vi "BRig_RT__Case_Exp__State_start__sendExpData_saveData.vi"(10 "input_dataLC":u16[](array[numeric]), 11 "input_dataExp":u16[](array[numeric])) -> ()   [LabVIEW 2014]
uses:
  <vilib>/Utility/file.llb/Write To Spreadsheet File (DBL).vi
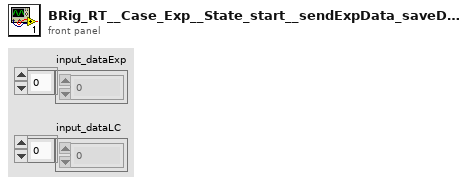
[diagram p1: front panel]
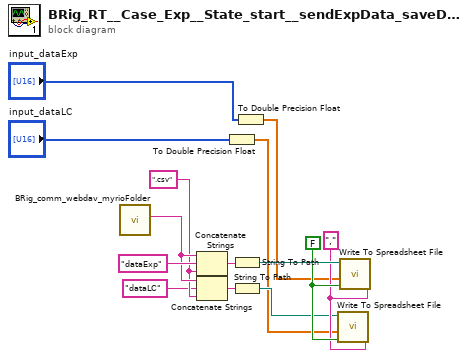
[diagram p0: block diagram]
diagram:
  w6 = "," ("delimiter (\\t)")
  w7 = FALSE ("append to file? (new file:F)")
  w10 = ".csv" ("string")
  n1 = call "BRig_comm_webdav_myrioFolder.vi"() -> ("output_myrioFolder"=w11:string)  [unwired: 11 in]
  n2 = Concatenate Strings(w11, "dataExp" ("input_filename"), w10) -> (w14:string)
  n3 = Concatenate Strings(w11, "dataLC" ("input_filename"), w10) -> (w8:string)
  n4 = To Double Precision Float(number="input_dataLC") -> (double precision float=w4:dbl[])
  n5 = String To Path(string=w14) -> (path=w12:path)
  n6 = String To Path(string=w8) -> (path=w5:path)
  n7 = To Double Precision Float(number="input_dataExp") -> (double precision float=w3:dbl[])
  n8 = call-poly <vilib>:"Write To Spreadsheet File.vi"("delimiter (\\t)"=w6, "append to file? (new file:F)"=w7, "1D data"=w4, "file path (dialog if empty)"=w5) -> ()  [unwired: 4 in, 1 out]
  n9 = call-poly <vilib>:"Write To Spreadsheet File.vi"("delimiter (\\t)"=w6, "append to file? (new file:F)"=w7, "1D data"=w3, "file path (dialog if empty)"=w12) -> ()  [unwired: 4 in, 1 out]
